vi "Emballage_BDD_GPAO_V_ARTICLE_DEStoINDEX.vi"(8 "error in (no error)":errorcluster, 11 "designation":string) -> (0 "error out":errorcluster, 1 "INDICE_REV":string, 2 "id_article":string, 3 "données":string[][](array[string]), 4 "pce_non_annule":bool, 5 "NB_PIECE_EMB":string)   [LabVIEW 2020]
uses:
  Modules/FS/60_FS_Controles/60_FS_SetGet.ctl
  <vilib>/addons/database/Connection.llb/DB Tools Open Connec (Path).vi
  <vilib>/addons/database/Connection.llb/Conn Execute.vi
  <vilib>/addons/database/Recordset.llb/Rec Fetch Recordset Data (R).vi
  <vilib>/addons/database/Recordset.llb/Rec Destroy - Connection.vi
  <vilib>/addons/database/NI_Database_API.lvlib
panel:
  out "ENR_ANNULE":string
  out "données 2":string[][](array[string])
  in  "Liste multicolonne":i32(listbox)
  out "columns 2":string[](array[string])
  out "Requète":string
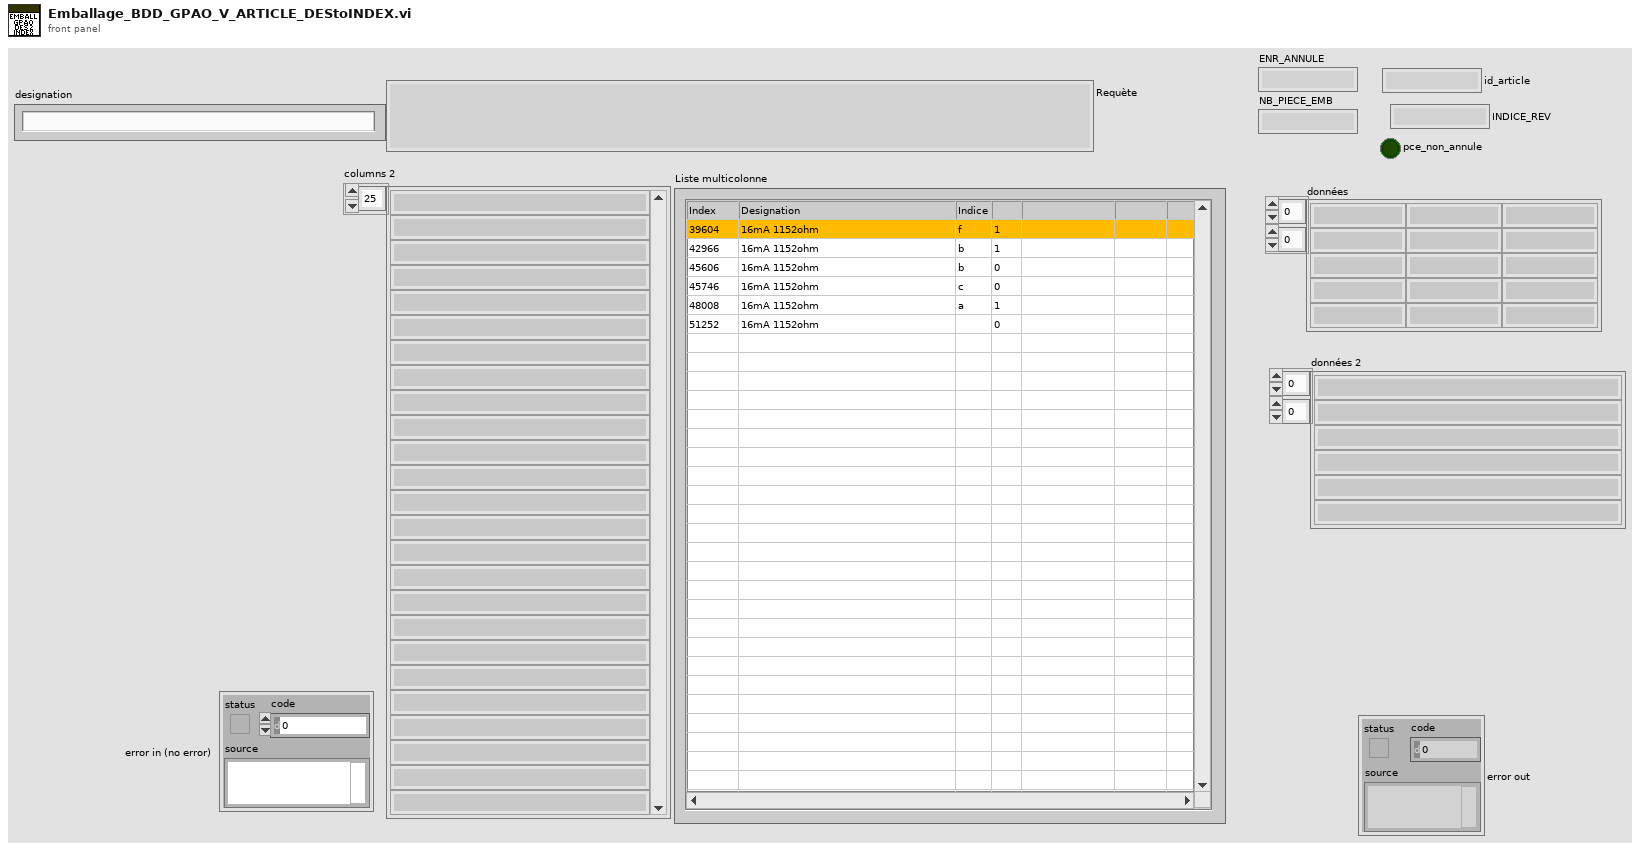
[diagram p1: front panel]
types:
  T1 = typedef "60_FS_SetGet.ctl" = enum16{"set", "get"}
  T2 = typedef "60_FS_CLT_Chemins.ctl" = cluster{"Racine_local":path, "Racine_reseau":path, "Racine_Support_Application":path, "Fichier_Journalisation":path, "Connexion_BDD_VSX":path, "Connexion_BDD_PLZ":path}
  T3 = typedef "NI_Database_API.lvlib/Conn ObjectReference.ctl" = refnum<k1>
  T4 = typedef "NI_Database_API.lvlib/Rec ObjectReference.ctl" = refnum<k1>
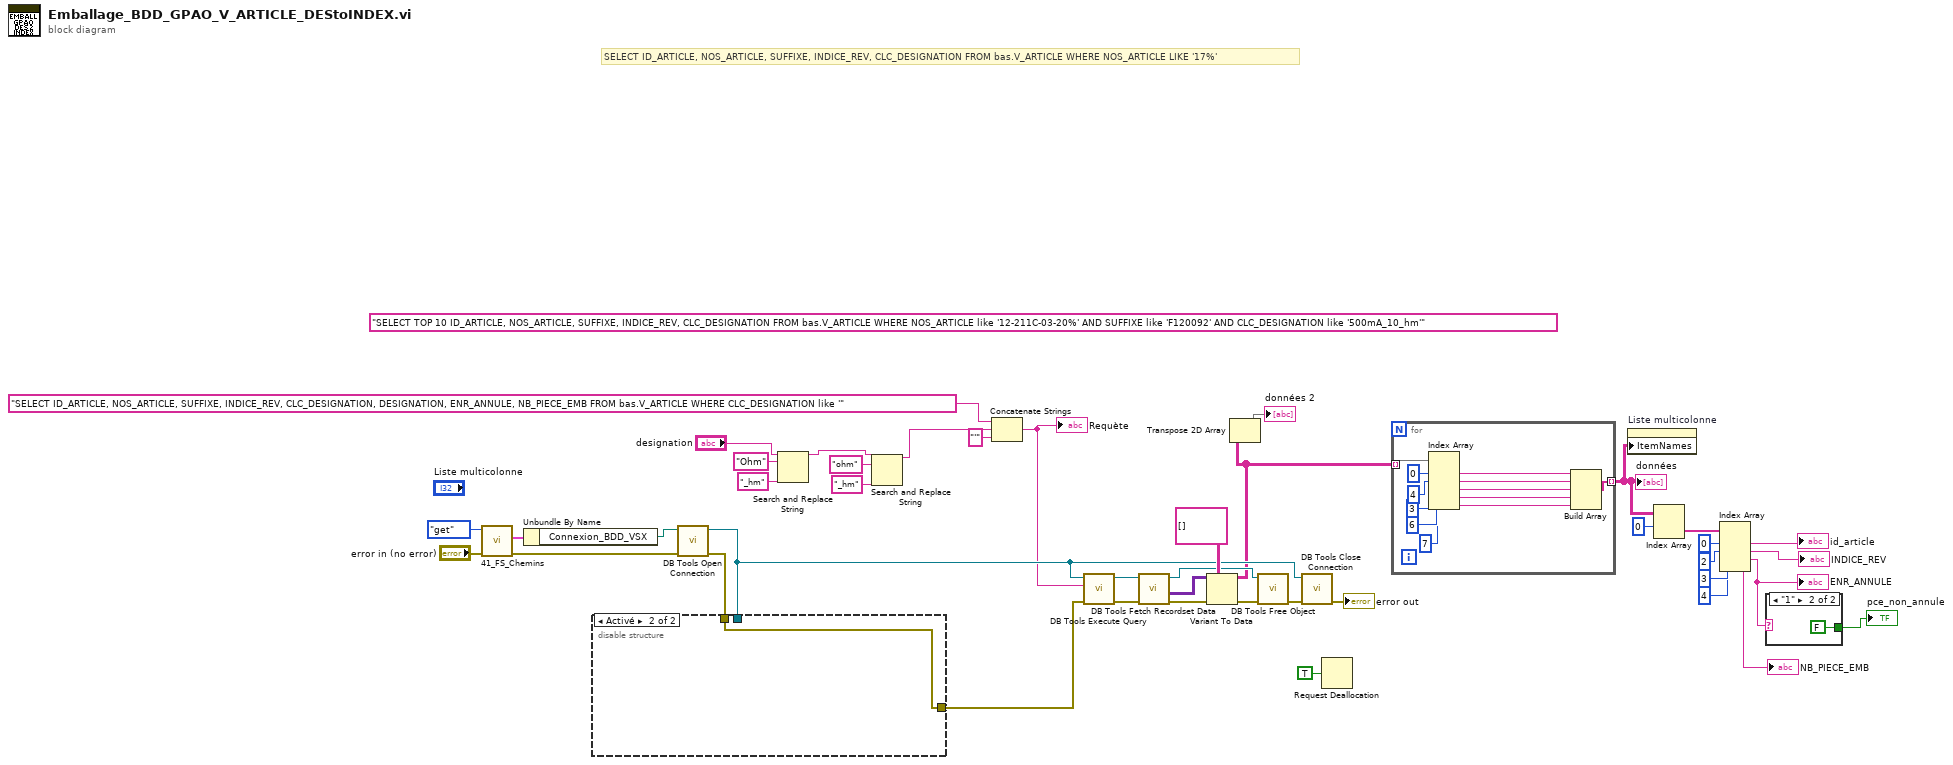
[diagram p0: block diagram]
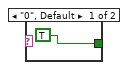
[diagram p2: hidden frame]
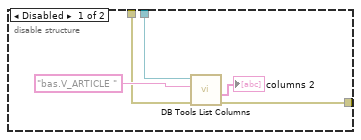
[diagram p3: hidden frame]
diagram:
  (unwired) "SELECT TOP 10 ID_ARTICLE, NOS_ARTICLE, SUFFIXE, INDICE_REV, CLC_DESIGNATION FROM bas.V_ARTICLE WHERE NOS_ARTICLE like '12-211C-03-20%' AND SUFFIXE like 'F120092' AND CLC_DESIGNATION like '500mA_10_hm'" ("Requète")
  # "SELECT ID_ARTICLE, NOS_ARTICLE, SUFFIXE, INDICE_REV, CLC_DESIGNATION FROM bas.V_ARTICLE WHERE NOS_ARTICLE LIKE '17%'"
  n1 = call "41_FS_Chemins.vi"("error in (no error)"="error in (no error)", "SetGet"=60_FS_SetGet."get") -> ("error out"=w40:errorcluster, "CLT_Chemins_out"=w41:T2)  [unwired: 8 in]
  n2 = Unbundle By Name(w41) -> ("Connexion_BDD_VSX"=w29:path)
  n3 = call-poly <vilib>:"DB Tools Open Connection.vi"("error in (no error)"=w40, "connection information"=w29) -> ("error out"=w27:errorcluster, "connection reference"=w28:T3)  [unwired: 6 in]
  n4 = disable-structure shown="Activé" {
    disable-tunnel: w28 -> [w47 _]
    disable-tunnel: w27 -> [w44 w48]
    disable-tunnel: [w43 w48] -> w26
    frame Disabled {
      n5 = call <vilib>:"DB Tools List Columns.vi"("error in (no error)"=w44, "table"="bas.V_ARTICLE " ("Table"), "connection reference"=w47) -> ("error out"=w43:errorcluster, "columns"=→"columns 2":string[])  [unwired: 1 in, 2 out]
    }
    frame Enabled {
    }
  }
  n6 = Search and Replace String(input string="designation", search string="Ohm" ("chaîne recherchée"), replace string="_hm" ("chaîne de remplacement (\"\")")) -> (result string=w8:string)  [unwired: 5 in, 3 out]
  n7 = Search and Replace String(input string=w8, search string="ohm" ("chaîne recherchée"), replace string="_hm" ("chaîne de remplacement (\"\")")) -> (result string=w7:string)  [unwired: 5 in, 3 out]
  n8 = Concatenate Strings("SELECT ID_ARTICLE, NOS_ARTICLE, SUFFIXE, INDICE_REV, CLC_DESIGNATION, DESIGNATION, ENR_ANNULE, NB_PIECE_EMB FROM bas.V_ARTICLE WHERE CLC_DESIGNATION like '" ("Requète"), w7, "'" ("chaîne")) -> (w22:string)
  "Requète" <- w22
  n9 = call-poly <vilib>:"DB Tools Execute Query.vi"("error in (no error)"=w26, "SQL query"=w22, "connection reference"=w28) -> ("error out"=w39:errorcluster, "recordset reference"=w38:T4)  [unwired: 5 in]
  n10 = call-poly <vilib>:"DB Tools Fetch Recordset Data.vi"("error in (no error)"=w39, "recordset reference"=w38) -> ("error out"=w35:errorcluster, "recordset data"=w36:variant[][], "recordset reference out"=w31:T4)  [unwired: 3 in]
  n11 = Variant To Data(error in=w35, type=string[][] [] ("Chaînes []"), Variant=w36) -> (data=w24:string[][], error out=w32:errorcluster)
  n12 = Transpose 2D Array(2D array=w24) -> (transposed array=→"données 2":string[][])
  n13 = call-poly <vilib>:"DB Tools Free Object.vi"("error in (no error)"=w32, "recordset reference"=w31) -> ("error out"=w30:errorcluster)  [unwired: 8 in, 1 out]
  n14 = call <vilib>:"DB Tools Close Connection.vi"("error in (no error)"=w30, "connection reference"=w28) -> ("error out"=→"error out":errorcluster)  [unwired: 5 in]
  n15 = Request Deallocation(TRUE ("flag")) -> ()
  n16 = for {
    tunnel: w24 -> [w60] mode=indexing
    tunnel: [w58] -> w21 mode=indexing
    n17 = Index Array(array=w60, index #1=0 ("indice"), index #2=4 ("indice"), index #3=3 ("indice"), index #4=6 ("indice"), index #5=7 ("indice")) -> (element #1=w59:string, element #2=w55:string, element #3=w53:string, element #4=w51:string, element #5=w49:string)
    n18 = Build Array(w59, w55, w53, w51, w49) -> (w58:string[])
  }
  "données" <- w21
  n19 = property on="Liste multicolonne" class="MCListbox (strict)"("ItemNames"=w21) -> ()  [unwired: 2 in, 2 out]
  n20 = Index Array(array=w21, index (row)=0 ("indice (ligne)")) -> (element=w19:string[])  [unwired: 1 in]
  n21 = Index Array(array=w19, index #1=0 ("indice"), index #2=2 ("indice"), index #3=3 ("indice"), index #4=4 ("indice")) -> (element #1=→"id_article":string, element #2=→"INDICE_REV":string, element #3=w3:string, element #4=→"NB_PIECE_EMB":string)
  "ENR_ANNULE" <- w3
  n22 = case shown="\"1\"" w3 {
    tunnel: [TRUE FALSE] -> w5
    frame "0", Default {
    }
    frame "1" {
    }
  }
  "pce_non_annule" <- w5
